vi "BRig_dataTrial_T_Reward.vi"() -> (2 "output_T_Reward":i32)   [LabVIEW 2014]
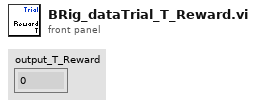
[diagram p1: front panel]
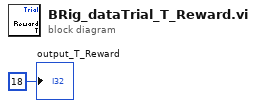
[diagram p0: block diagram]
diagram:
  "output_T_Reward" <- 18 ("output_iBlock")
